vi "Main A.vi"() -> ()   [LabVIEW 2025]
uses:
  numindicator.ctl
  <vilib>/numeric/Random Number (Range) U64.vi
  <vilib>/numeric/Random Number (Range) I64.vi
  <vilib>/numeric/sub_Random U32.vi
panel:
  out "Speed":dbl
  in  "RESET":bool
  out "Table of slot elements":u16[][](array[numeric])
  in  "stop":bool
  out "LED 12":bool
  out "LED 11":bool
  out "LED 10":bool
  out "LED 7":bool
  out "LED 8":bool
  out "LED 9":bool
  out "LED 3":bool
  out "LED 2":bool
  out "LED 1":bool
  out "LED 4":bool
  out "LED 5":bool
  out "LED 6":bool
  out "Ring 9":u16(ring)
  out "Ring 8":u16(ring)
  out "Ring 7":u16(ring)
  out "Ring 6":u16(ring)
  out "Ring 5":u16(ring)
  out "Ring 4":u16(ring)
  out "Ring 3":u16(ring)
  out "Ring 2":u16(ring)
  out "Ring":u16(ring)
  in  "add credit":bool
  out "String":string
  out "last win":T1
  out "wallet":T1
  in  "bet":dbl step=10.0
  in  "spin":bool
  # "WALLET"
  # "PLACE BET"
  # "LAST WIN"
  # "DEBUG MENU"
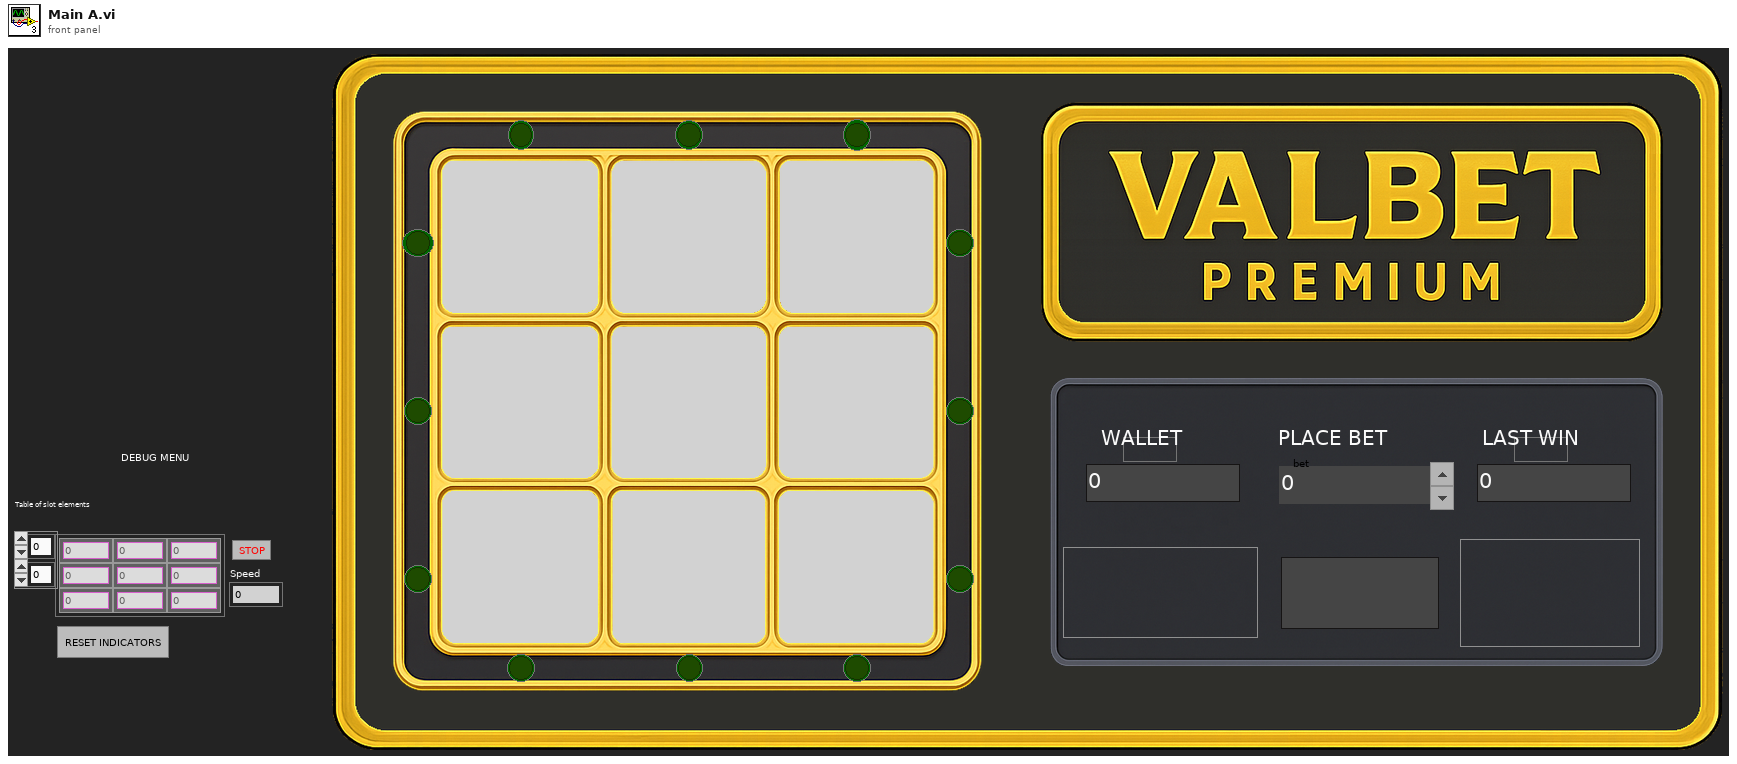
[diagram p1: front panel]
types:
  T1 = typedef "numindicator.ctl" = dbl
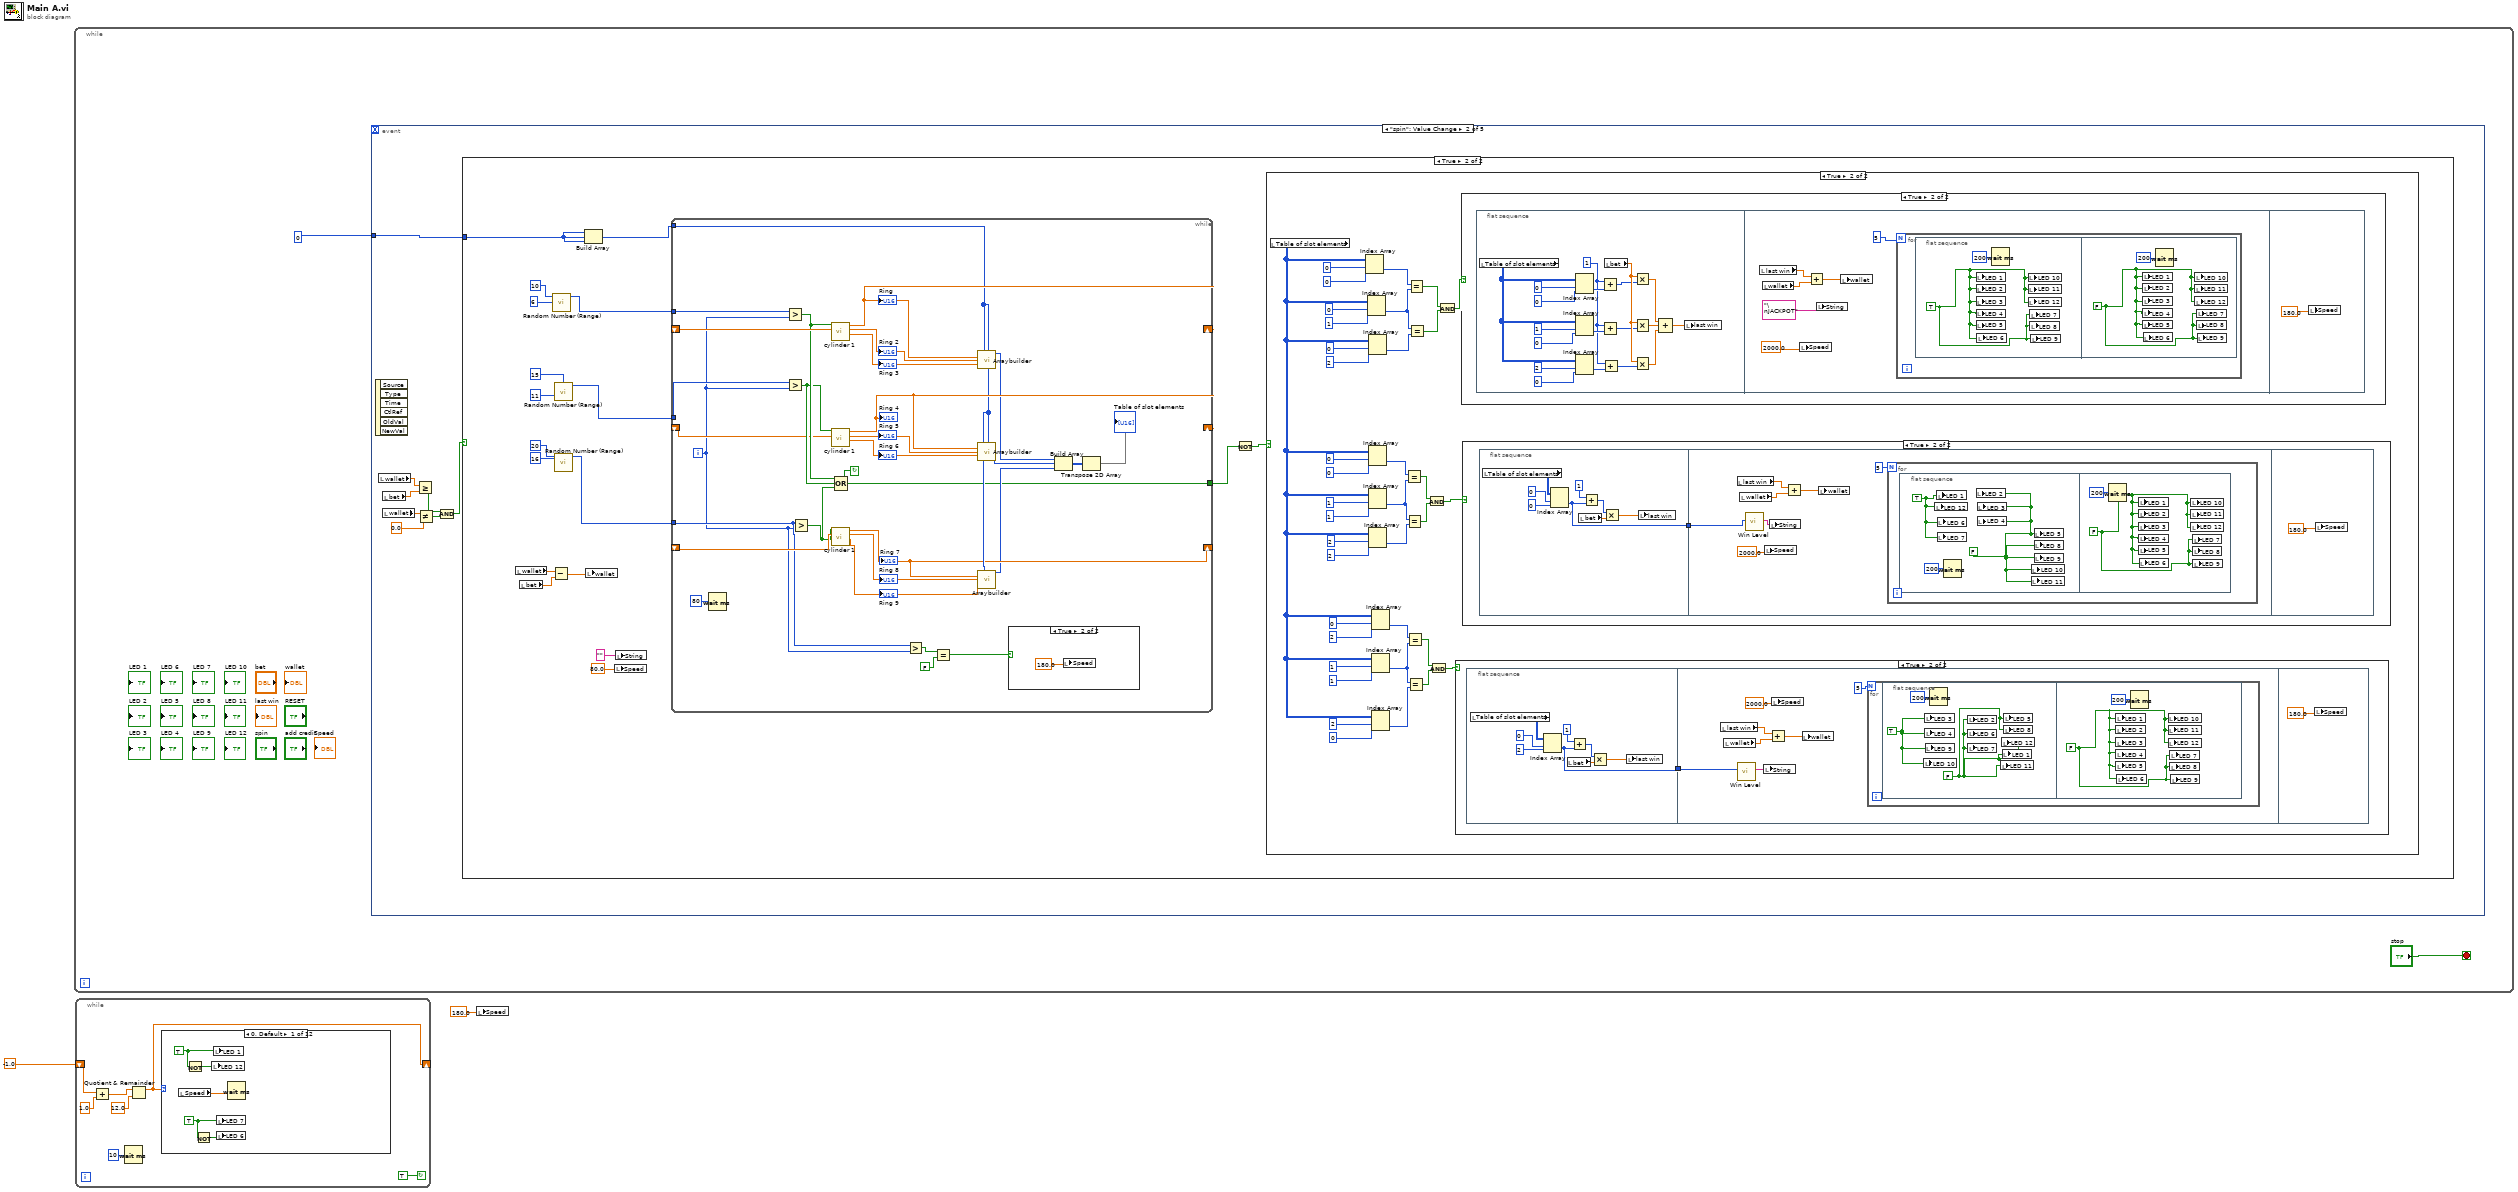
[diagram p0: block diagram]
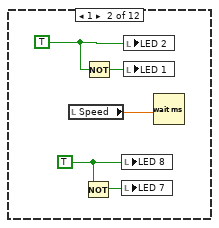
[diagram p2: hidden frame]
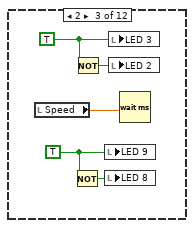
[diagram p3: hidden frame]
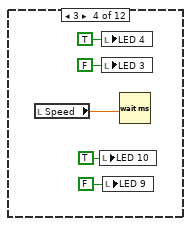
[diagram p4: hidden frame]
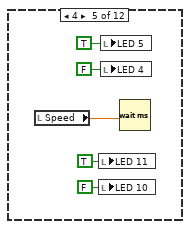
[diagram p5: hidden frame]
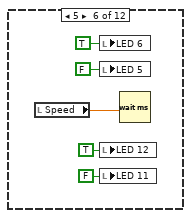
[diagram p6: hidden frame]
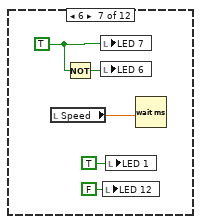
[diagram p7: hidden frame]
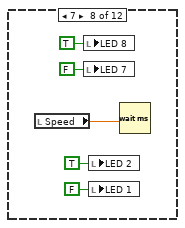
[diagram p8: hidden frame]
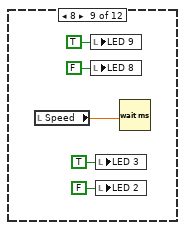
[diagram p9: hidden frame]
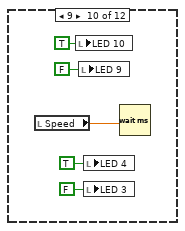
[diagram p10: hidden frame]
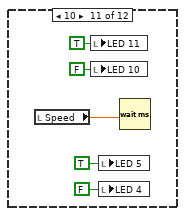
[diagram p11: hidden frame]
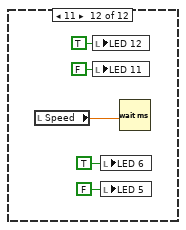
[diagram p12: hidden frame]
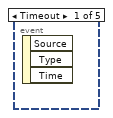
[diagram p13: hidden frame]
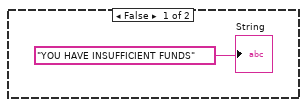
[diagram p14: hidden frame]
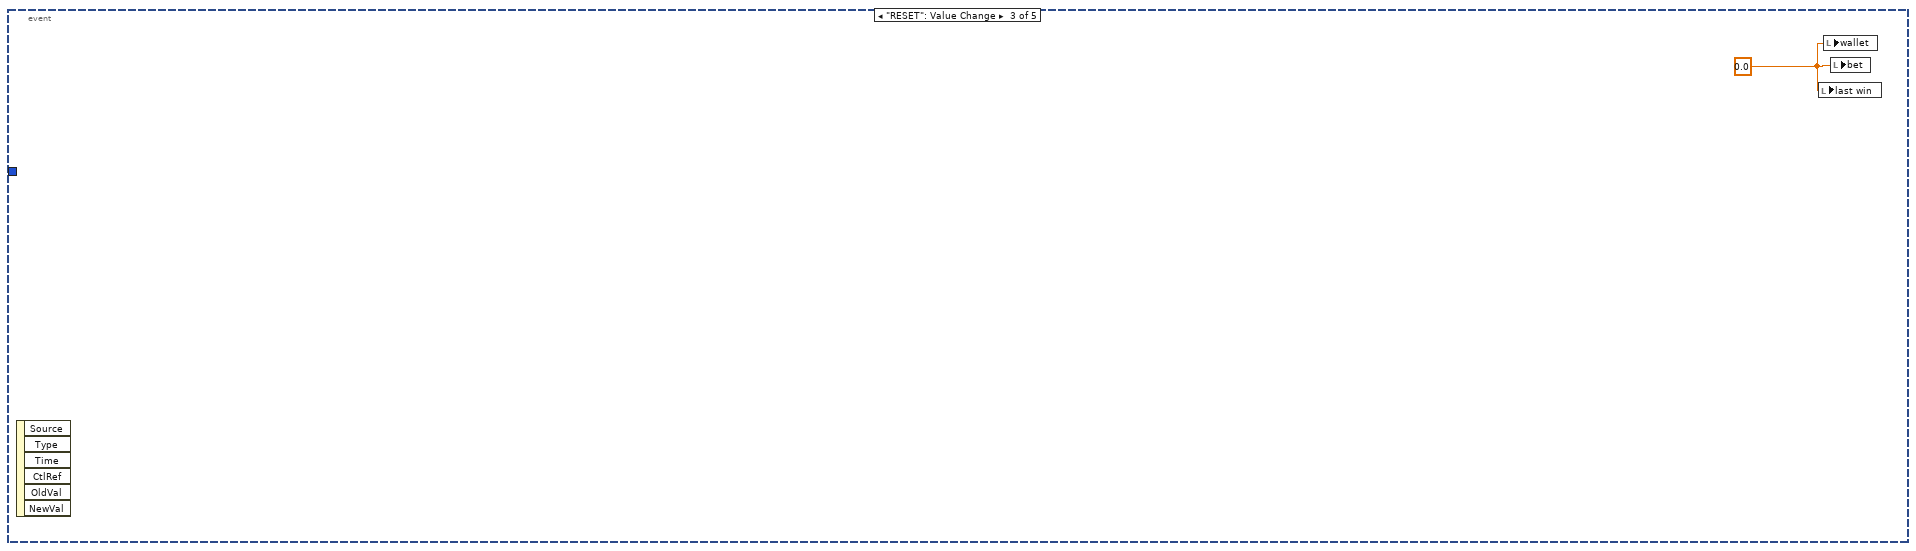
[diagram p20: hidden frame]
diagram:
  n1 = while {
    stop <- "stop" stop-if-true
    n2 = event shown="[1] \"spin\": Value Change" {
      selector: _ -> [_ _ _ _ _]
      dyn-events: _ -> [_ _ _ _ _]
      timeout: _ -> [_ _ _ _ _]
      tunnel: 0 -> [_ w12 _ _ _]
      event Timeout {
        n3 = event-data() -> ()  [unwired: 1 in, 3 out]
      }
      event "spin": Value Change {
        n4 = event-data() -> ()  [unwired: 1 in, 6 out]
        n5 = local read "wallet"() -> (w10:T1)
        n6 = local read "bet"() -> (w11:dbl)
        n7 = local read "wallet"() -> (w9:T1)
        n8 = Greater Or Equal?(x=w10, y=w11) -> (x >= y?=w6:bool)
        n9 = Not Equal?(x=w9, y=T1 0.0) -> (x != y?=w5:bool)
        n10 = Compound Arithmetic op=AND(w6, w5) -> (w7:bool)
        n11 = case shown="True" w7 {
          tunnel: w12 -> [_ w20]
          frame False {
            "String" <- "YOU HAVE INSUFFICIENT FUNDS"
          }
          frame True {
            n12 = local read "wallet"() -> (w19:T1)
            n13 = local read "bet"() -> (w17:dbl)
            n14 = Subtract(x=w19, y=w17) -> (x-y=w18:T1)
            n15 = call-poly <vilib>:"Random Number (Range).vi"("lower bound (-100)"=i64 6, "upper bound (100)"=i64 10) -> ("number"=w30:i64)  [unwired: 9 in]
            n16 = call-poly <vilib>:"Random Number (Range).vi"("lower bound (0)"=u64 11, "upper bound (100)"=u64 15) -> ("number"=w31:u64)  [unwired: 9 in]
            n17 = call-poly <vilib>:"Random Number (Range).vi"("lower bound (0)"=u64 16, "upper bound (100)"=u64 20) -> ("number"=w16:u64)  [unwired: 9 in]
            n18 = Build Array(w20, w20, w20) -> (w21:i32[])
            n19 = local write "wallet"(w18) -> ()
            n20 = local write "Speed"(80.0 ("Variable 2")) -> ()
            n21 = local write "String"("") -> ()
            n22 = while {
              tunnel: w30 -> [w172]
              tunnel: w31 -> [w171]
              tunnel: w16 -> [w147]
              shift-right: [w160] -> _
              shift-left: _ -> [w166]
              shift-right: [w156] -> _
              shift-left: _ -> [w165]
              shift-right: [w161] -> _
              shift-left: _ -> [w170]
              tunnel: [w148] -> w23
              tunnel: w21 -> [w157]
              i -> [w146]
              stop <- w148 continue-if-true
              n23 = Wait (ms)(milliseconds to wait=80) -> ()  [unwired: 1 out]
              n24 = Greater?(x=w172, y=w146) -> (0:w168:bool)
              n25 = Greater?(x=w171, y=w146) -> (0:w167:bool)
              n26 = Greater?(x=w147, y=w146) -> (0:w164:bool)
              n27 = call "cylinder 1.vi"("Element value"=w170, "Boolean"=w168) -> ("Element 3"=w163:dbl, "Element 2"=w162:dbl, "Element 1"=w161:dbl)  [unwired: 7 in]
              "Ring" <- w161
              "Ring 2" <- w162
              "Ring 3" <- w163
              n28 = call "cylinder 1.vi"("Element value"=w166, "Boolean"=w167) -> ("Element 3"=w158:dbl, "Element 2"=w159:dbl, "Element 1"=w160:dbl)  [unwired: 7 in]
              "Ring 4" <- w160
              "Ring 5" <- w159
              "Ring 6" <- w158
              n29 = call "cylinder 1.vi"("Element value"=w165, "Boolean"=w164) -> ("Element 3"=w154:dbl, "Element 2"=w155:dbl, "Element 1"=w156:dbl)  [unwired: 7 in]
              "Ring 7" <- w156
              "Ring 8" <- w155
              "Ring 9" <- w154
              n30 = Compound Arithmetic op=OR(w168, w167, w164) -> (w148:bool)
              n31 = Greater?(x=w147, y=w146) -> (0:w145:bool)
              n32 = Equal?(x=w145, y=FALSE) -> (x = y?=w143:bool)
              n33 = call "Arraybuilder.vi"("Array in"=w157, "Element 1"=w161, "Element 2"=w162, "Element 3"=w163) -> ("Array out"=w151:u16[])  [unwired: 11 in]
              n34 = call "Arraybuilder.vi"("Array in"=w157, "Element 1"=w160, "Element 2"=w159, "Element 3"=w158) -> ("Array out"=w152:u16[])  [unwired: 11 in]
              n35 = call "Arraybuilder.vi"("Array in"=w157, "Element 1"=w156, "Element 2"=w155, "Element 3"=w154) -> ("Array out"=w153:u16[])  [unwired: 11 in]
              n36 = case shown="True" w143 {
                frame False {
                }
                frame True {
                  n37 = local write "Speed"(180.0) -> ()
                }
              }
              n38 = Build Array(w151, w152, w153) -> (w150:u16[][])
              n39 = Transpose 2D Array(2D array=w150) -> (transposed array=→"Table of slot elements":u16[][])
            }
            n40 = Not(x=w23) -> (.not. x?=w22:bool)
            n41 = case shown="True" w22 {
              frame False {
              }
              frame True {
                n42 = local read "Table of slot elements"() -> (w50:u16[][])
                n43 = Index Array(array=w50, index (row)=0, index (col)=0 ("index (row)")) -> (element=w49:u16)
                n44 = Index Array(array=w50, index (row)=0, index (col)=1 ("index (row)")) -> (element=w47:u16)
                n45 = Index Array(array=w50, index (row)=0, index (col)=2 ("index (row)")) -> (element=w48:u16)
                n46 = Index Array(array=w50, index (row)=0, index (col)=0 ("index (row)")) -> (element=w36:u16)
                n47 = Index Array(array=w50, index (row)=1, index (col)=1 ("index (row)")) -> (element=w35:u16)
                n48 = Index Array(array=w50, index (row)=2, index (col)=2 ("index (row)")) -> (element=w37:u16)
                n49 = Index Array(array=w50, index (row)=0, index (col)=2 ("index (row)")) -> (element=w38:u16)
                n50 = Index Array(array=w50, index (row)=1, index (col)=1 ("index (row)")) -> (element=w39:u16)
                n51 = Index Array(array=w50, index (row)=2, index (col)=0 ("index (row)")) -> (element=w40:u16)
                n52 = Equal?(x=w36, y=w35) -> (x = y?=w43:bool)
                n53 = Equal?(x=w35, y=w37) -> (x = y?=w44:bool)
                n54 = Equal?(x=w38, y=w39) -> (x = y?=w42:bool)
                n55 = Equal?(x=w39, y=w40) -> (x = y?=w41:bool)
                n56 = Equal?(x=w49, y=w47) -> (x = y?=w46:bool)
                n57 = Equal?(x=w47, y=w48) -> (x = y?=w45:bool)
                n58 = And(x=w43, y=w44) -> (x .and. y?=w33:bool)
                n59 = And(x=w42, y=w41) -> (x .and. y?=w34:bool)
                n60 = And(x=w46, y=w45) -> (x .and. y?=w32:bool)
                n61 = case shown="True" w34 {
                  frame False {
                  }
                  frame True {
                    n62 = flat-sequence {
                      tunnel: [w70] -> w69
                      tunnel: w69 -> [w80]
                      frame #0 {
                        n63 = local read "Table of slot elements"() -> (w77:u16[][])
                        n64 = Index Array(array=w77, index (row)=0, index (col)=2 ("index (row)")) -> (element=w70:u16)
                        n65 = local read "bet"() -> (w73:dbl)
                        n66 = Add(x=1 ("index (row)"), y=w70) -> (x+y=w72:i32)
                        n67 = Multiply(x=w72, y=w73) -> (x*y=w71:dbl)
                        n68 = local write "last win"(w71) -> ()
                      }
                      frame #1 {
                        n69 = local read "last win"() -> (w83:T1)
                        n70 = local read "wallet"() -> (w82:T1)
                        n71 = call "Win Level.vi"("icon strength"=w80) -> ("String"=w81:string)  [unwired: 10 in]
                        n72 = local write "String"(w81) -> ()
                        n73 = Add(x=w83, y=w82) -> (x+y=w84:T1)
                        n74 = local write "Speed"(2000.0) -> ()
                        n75 = local write "wallet"(w84) -> ()
                        n76 = for {
                          N: 5 -> [_]
                          n77 = flat-sequence {
                            frame #0 {
                              w87 = FALSE ("LED 1")
                              w86 = TRUE ("LED 1")
                              n78 = local write "LED 10"(w86) -> ()
                              n79 = local write "LED 3"(w86) -> ()
                              n80 = local write "LED 4"(w86) -> ()
                              n81 = local write "LED 9"(w86) -> ()
                              n82 = Wait (ms)(milliseconds to wait=u32 200) -> ()  [unwired: 1 out]
                              n83 = local write "LED 2"(w87) -> ()
                              n84 = local write "LED 6"(w87) -> ()
                              n85 = local write "LED 7"(w87) -> ()
                              n86 = local write "LED 11"(w87) -> ()
                              n87 = local write "LED 12"(w87) -> ()
                              n88 = local write "LED 1"(w87) -> ()
                              n89 = local write "LED 5"(w87) -> ()
                              n90 = local write "LED 8"(w87) -> ()
                            }
                            frame #1 {
                              w89 = FALSE ("LED 1")
                              n91 = local write "LED 1"(w89) -> ()
                              n92 = local write "LED 2"(w89) -> ()
                              n93 = local write "LED 3"(w89) -> ()
                              n94 = local write "LED 4"(w89) -> ()
                              n95 = local write "LED 5"(w89) -> ()
                              n96 = local write "LED 6"(w89) -> ()
                              n97 = Wait (ms)(milliseconds to wait=u32 200) -> ()  [unwired: 1 out]
                              n98 = local write "LED 10"(w89) -> ()
                              n99 = local write "LED 11"(w89) -> ()
                              n100 = local write "LED 12"(w89) -> ()
                              n101 = local write "LED 7"(w89) -> ()
                              n102 = local write "LED 8"(w89) -> ()
                              n103 = local write "LED 9"(w89) -> ()
                            }
                          }
                        }
                      }
                      frame #2 {
                        n104 = local write "Speed"(180.0) -> ()
                      }
                    }
                  }
                }
                n105 = case shown="True" w32 {
                  frame False {
                  }
                  frame True {
                    n106 = flat-sequence {
                      frame #0 {
                        w116 = u16 1 ("x")
                        n107 = local read "Table of slot elements"() -> (w131:u16[][])
                        n108 = Index Array(array=w131, index (row)=0, index (col)=0 ("index (row)")) -> (element=w117:u16)
                        n109 = Index Array(array=w131, index (row)=1, index (col)=0 ("index (row)")) -> (element=w119:u16)
                        n110 = Index Array(array=w131, index (row)=2, index (col)=0 ("index (row)")) -> (element=w118:u16)
                        n111 = Add(x=w116, y=w117) -> (x+y=w114:u16)
                        n112 = Add(x=w116, y=w119) -> (x+y=w115:u16)
                        n113 = Add(x=w116, y=w118) -> (x+y=w113:u16)
                        n114 = local read "bet"() -> (w124:dbl)
                        n115 = Multiply(x=w124, y=w114) -> (x*y=w122:dbl)
                        n116 = Multiply(x=w124, y=w115) -> (x*y=w121:dbl)
                        n117 = Multiply(x=w124, y=w113) -> (x*y=w120:dbl)
                        n118 = Compound Arithmetic op=ADD(w122, w121, w120) -> (w123:dbl)
                        n119 = local write "last win"(w123) -> ()
                      }
                      frame #1 {
                        n120 = local read "last win"() -> (w135:T1)
                        n121 = local read "wallet"() -> (w136:T1)
                        n122 = local write "Speed"(2000.0) -> ()
                        n123 = Add(x=w135, y=w136) -> (x+y=w134:T1)
                        n124 = local write "String"("\nJACKPOT") -> ()
                        n125 = local write "wallet"(w134) -> ()
                        n126 = for {
                          N: 5 -> [_]
                          n127 = flat-sequence {
                            frame #0 {
                              w139 = TRUE ("LED 1")
                              n128 = local write "LED 1"(w139) -> ()
                              n129 = local write "LED 2"(w139) -> ()
                              n130 = local write "LED 3"(w139) -> ()
                              n131 = local write "LED 4"(w139) -> ()
                              n132 = local write "LED 5"(w139) -> ()
                              n133 = local write "LED 6"(w139) -> ()
                              n134 = Wait (ms)(milliseconds to wait=u32 200) -> ()  [unwired: 1 out]
                              n135 = local write "LED 10"(w139) -> ()
                              n136 = local write "LED 11"(w139) -> ()
                              n137 = local write "LED 12"(w139) -> ()
                              n138 = local write "LED 7"(w139) -> ()
                              n139 = local write "LED 8"(w139) -> ()
                              n140 = local write "LED 9"(w139) -> ()
                            }
                            frame #1 {
                              w141 = FALSE ("LED 1")
                              n141 = local write "LED 1"(w141) -> ()
                              n142 = local write "LED 2"(w141) -> ()
                              n143 = local write "LED 3"(w141) -> ()
                              n144 = local write "LED 4"(w141) -> ()
                              n145 = local write "LED 5"(w141) -> ()
                              n146 = local write "LED 6"(w141) -> ()
                              n147 = Wait (ms)(milliseconds to wait=u32 200) -> ()  [unwired: 1 out]
                              n148 = local write "LED 10"(w141) -> ()
                              n149 = local write "LED 11"(w141) -> ()
                              n150 = local write "LED 12"(w141) -> ()
                              n151 = local write "LED 7"(w141) -> ()
                              n152 = local write "LED 8"(w141) -> ()
                              n153 = local write "LED 9"(w141) -> ()
                            }
                          }
                        }
                      }
                      frame #2 {
                        n154 = local write "Speed"(180.0) -> ()
                      }
                    }
                  }
                }
                n155 = case shown="True" w33 {
                  frame False {
                  }
                  frame True {
                    n156 = flat-sequence {
                      tunnel: [w92] -> w91
                      tunnel: w91 -> [w102]
                      frame #0 {
                        n157 = local read "Table of slot elements"() -> (w99:u16[][])
                        n158 = Index Array(array=w99, index (row)=0, index (col)=0 ("index (row)")) -> (element=w92:u16)
                        n159 = local read "bet"() -> (w95:dbl)
                        n160 = Add(x=1 ("index (row)"), y=w92) -> (x+y=w94:i32)
                        n161 = Multiply(x=w94, y=w95) -> (x*y=w93:dbl)
                        n162 = local write "last win"(w93) -> ()
                      }
                      frame #1 {
                        n163 = local read "last win"() -> (w104:T1)
                        n164 = local read "wallet"() -> (w103:T1)
                        n165 = call "Win Level.vi"("icon strength"=w102) -> ("String"=w101:string)  [unwired: 10 in]
                        n166 = local write "Speed"(2000.0) -> ()
                        n167 = local write "String"(w101) -> ()
                        n168 = Add(x=w104, y=w103) -> (x+y=w105:T1)
                        n169 = local write "wallet"(w105) -> ()
                        n170 = for {
                          N: 5 -> [_]
                          n171 = flat-sequence {
                            frame #0 {
                              w109 = FALSE ("LED 1")
                              w108 = TRUE ("LED 1")
                              n172 = local write "LED 12"(w108) -> ()
                              n173 = local write "LED 1"(w108) -> ()
                              n174 = local write "LED 6"(w108) -> ()
                              n175 = local write "LED 7"(w108) -> ()
                              n176 = Wait (ms)(milliseconds to wait=u32 200) -> ()  [unwired: 1 out]
                              n177 = local write "LED 2"(w109) -> ()
                              n178 = local write "LED 3"(w109) -> ()
                              n179 = local write "LED 4"(w109) -> ()
                              n180 = local write "LED 10"(w109) -> ()
                              n181 = local write "LED 11"(w109) -> ()
                              n182 = local write "LED 5"(w109) -> ()
                              n183 = local write "LED 8"(w109) -> ()
                              n184 = local write "LED 9"(w109) -> ()
                            }
                            frame #1 {
                              w111 = FALSE ("LED 1")
                              n185 = Wait (ms)(milliseconds to wait=u32 200) -> ()  [unwired: 1 out]
                              n186 = local write "LED 1"(w111) -> ()
                              n187 = local write "LED 2"(w111) -> ()
                              n188 = local write "LED 3"(w111) -> ()
                              n189 = local write "LED 4"(w111) -> ()
                              n190 = local write "LED 5"(w111) -> ()
                              n191 = local write "LED 6"(w111) -> ()
                              n192 = local write "LED 10"(w111) -> ()
                              n193 = local write "LED 11"(w111) -> ()
                              n194 = local write "LED 12"(w111) -> ()
                              n195 = local write "LED 7"(w111) -> ()
                              n196 = local write "LED 8"(w111) -> ()
                              n197 = local write "LED 9"(w111) -> ()
                            }
                          }
                        }
                      }
                      frame #2 {
                        n198 = local write "Speed"(180.0) -> ()
                      }
                    }
                  }
                }
              }
            }
          }
        }
      }
      event "RESET": Value Change {
        w174 = 0.0
        n199 = event-data() -> ()  [unwired: 1 in, 6 out]
        n200 = local write "last win"(w174) -> ()
        n201 = local write "wallet"(w174) -> ()
        n202 = local write "bet"(w174) -> ()
      }
      event "add credit": Value Change {
        n203 = event-data() -> ()  [unwired: 1 in, 6 out]
        n204 = local read "wallet"() -> (w177:T1)
        n205 = Add(x=w177, y=T1 1000.0) -> (x+y=w176:T1)
        n206 = local write "wallet"(w176) -> ()
      }
      event "bet": Value Change {
        n207 = event-data() -> ()  [unwired: 1 in, 6 out]
        n208 = local read "bet"() -> (w179:dbl)
        n209 = Less?(x=w179, y=0.0) -> (x < y?=w178:bool)
        n210 = case shown="True" w178 {
          frame False {
          }
          frame True {
            n211 = local write "bet"(0.0 ("bet")) -> ()
            n212 = local write "String"("BET \nCANNOT BE \nNEGATIVE" ("String")) -> ()
          }
        }
      }
    }
  }
  n213 = while {
    shift-right: [w188] -> _
    shift-left: -1.0 -> [w187]
    stop <- TRUE continue-if-true
    n214 = Add(x=w187, y=1.0) -> (x+y=w186:dbl)
    n215 = Wait (ms)(milliseconds to wait=u32 10) -> ()  [unwired: 1 out]
    n216 = Quotient & Remainder(x=w186, y=12.0) -> (x-y*floor(x/y)=w188:dbl)  [unwired: 1 out]
    n217 = case shown="0, Default" w188 {
      frame 0, Default {
        w191 = TRUE ("LED 1")
        w192 = TRUE ("LED 1")
        n218 = local read "Speed"() -> (w194:dbl)
        n219 = Not(x=w192) -> (.not. x?=w193:bool)
        n220 = Not(x=w191) -> (.not. x?=w190:bool)
        n221 = local write "LED 12"(w193) -> ()
        n222 = local write "LED 1"(w192) -> ()
        n223 = local write "LED 7"(w191) -> ()
        n224 = local write "LED 6"(w190) -> ()
        n225 = Wait (ms)(milliseconds to wait=w194) -> ()  [unwired: 1 out]
      }
      frame 1 {
        w196 = TRUE ("LED 1")
        w198 = TRUE ("LED 1")
        n226 = local read "Speed"() -> (w199:dbl)
        n227 = Not(x=w196) -> (.not. x?=w195:bool)
        n228 = Not(x=w198) -> (.not. x?=w197:bool)
        n229 = local write "LED 8"(w196) -> ()
        n230 = local write "LED 7"(w195) -> ()
        n231 = local write "LED 2"(w198) -> ()
        n232 = local write "LED 1"(w197) -> ()
        n233 = Wait (ms)(milliseconds to wait=w199) -> ()  [unwired: 1 out]
      }
      frame 2 {
        w201 = TRUE ("LED 1")
        w203 = TRUE ("LED 1")
        n234 = local read "Speed"() -> (w204:dbl)
        n235 = Not(x=w201) -> (.not. x?=w200:bool)
        n236 = Not(x=w203) -> (.not. x?=w202:bool)
        n237 = local write "LED 9"(w201) -> ()
        n238 = local write "LED 8"(w200) -> ()
        n239 = local write "LED 3"(w203) -> ()
        n240 = local write "LED 2"(w202) -> ()
        n241 = Wait (ms)(milliseconds to wait=w204) -> ()  [unwired: 1 out]
      }
      frame 3 {
        n242 = local read "Speed"() -> (w209:dbl)
        n243 = local write "LED 10"(TRUE ("LED 1")) -> ()
        n244 = local write "LED 4"(TRUE ("LED 1")) -> ()
        n245 = local write "LED 3"(FALSE ("LED 4")) -> ()
        n246 = local write "LED 9"(FALSE ("LED 4")) -> ()
        n247 = Wait (ms)(milliseconds to wait=w209) -> ()  [unwired: 1 out]
      }
      frame 4 {
        n248 = local read "Speed"() -> (w214:dbl)
        n249 = local write "LED 11"(TRUE ("LED 1")) -> ()
        n250 = local write "LED 10"(FALSE ("LED 4")) -> ()
        n251 = local write "LED 5"(TRUE ("LED 1")) -> ()
        n252 = local write "LED 4"(FALSE ("LED 4")) -> ()
        n253 = Wait (ms)(milliseconds to wait=w214) -> ()  [unwired: 1 out]
      }
      frame 5 {
        n254 = local read "Speed"() -> (w219:dbl)
        n255 = local write "LED 6"(TRUE ("LED 1")) -> ()
        n256 = local write "LED 5"(FALSE ("LED 4")) -> ()
        n257 = local write "LED 12"(TRUE ("LED 1")) -> ()
        n258 = local write "LED 11"(FALSE ("LED 4")) -> ()
        n259 = Wait (ms)(milliseconds to wait=w219) -> ()  [unwired: 1 out]
      }
      frame 6 {
        w220 = TRUE ("LED 1")
        n260 = local read "Speed"() -> (w224:dbl)
        n261 = Not(x=w220) -> (.not. x?=w221:bool)
        n262 = local write "LED 7"(w220) -> ()
        n263 = local write "LED 6"(w221) -> ()
        n264 = local write "LED 12"(FALSE ("LED 4")) -> ()
        n265 = local write "LED 1"(TRUE ("LED 1")) -> ()
        n266 = Wait (ms)(milliseconds to wait=w224) -> ()  [unwired: 1 out]
      }
      frame 7 {
        n267 = local read "Speed"() -> (w229:dbl)
        n268 = local write "LED 8"(TRUE ("LED 1")) -> ()
        n269 = local write "LED 7"(FALSE ("LED 4")) -> ()
        n270 = local write "LED 2"(TRUE ("LED 1")) -> ()
        n271 = local write "LED 1"(FALSE ("LED 4")) -> ()
        n272 = Wait (ms)(milliseconds to wait=w229) -> ()  [unwired: 1 out]
      }
      frame 8 {
        n273 = local read "Speed"() -> (w234:dbl)
        n274 = local write "LED 9"(TRUE ("LED 1")) -> ()
        n275 = local write "LED 8"(FALSE ("LED 4")) -> ()
        n276 = local write "LED 3"(TRUE ("LED 1")) -> ()
        n277 = local write "LED 2"(FALSE ("LED 4")) -> ()
        n278 = Wait (ms)(milliseconds to wait=w234) -> ()  [unwired: 1 out]
      }
      frame 9 {
        n279 = local read "Speed"() -> (w239:dbl)
        n280 = local write "LED 10"(TRUE ("LED 1")) -> ()
        n281 = local write "LED 9"(FALSE ("LED 4")) -> ()
        n282 = local write "LED 4"(TRUE ("LED 1")) -> ()
        n283 = local write "LED 3"(FALSE ("LED 4")) -> ()
        n284 = Wait (ms)(milliseconds to wait=w239) -> ()  [unwired: 1 out]
      }
      frame 10 {
        n285 = local read "Speed"() -> (w244:dbl)
        n286 = local write "LED 11"(TRUE ("LED 1")) -> ()
        n287 = local write "LED 10"(FALSE ("LED 4")) -> ()
        n288 = local write "LED 5"(TRUE ("LED 1")) -> ()
        n289 = local write "LED 4"(FALSE ("LED 4")) -> ()
        n290 = Wait (ms)(milliseconds to wait=w244) -> ()  [unwired: 1 out]
      }
      frame 11 {
        n291 = local read "Speed"() -> (w249:dbl)
        n292 = local write "LED 12"(TRUE ("LED 1")) -> ()
        n293 = local write "LED 11"(FALSE ("LED 4")) -> ()
        n294 = local write "LED 6"(TRUE ("LED 1")) -> ()
        n295 = local write "LED 5"(FALSE ("LED 4")) -> ()
        n296 = Wait (ms)(milliseconds to wait=w249) -> ()  [unwired: 1 out]
      }
    }
  }
  n297 = local write "Speed"(180.0 ("Variable 2")) -> ()
